vi "mop&inc.vi"() -> ()   [LabVIEW 2017]
panel:
  in  "子面板传来-开始测试":bool
  out "设备编号 2":string
  out "测试方式 2":enum32{"手动测试", "自动测试"}(ring)
  out "连接ID":refnum<k5>
  out "网络连接指示":bool
  in  "每次数据量":i32
  out "当前时间":string
  out "用户":string
  out "设备编号":dbl
  out "测试编号":dbl
  out "测试类型":dbl
  out "测试批次":dbl
  # "测试信息"
  # "根据测试类型\n和手/自动；决定\n子面板显示manual\n和auto页。manual分\nmop-manual和\ninc-manual，各功能\n按钮就是各子模块。\nauto有\n测试项（子模块）\n配置选项页。"
  # "登录信息显示"
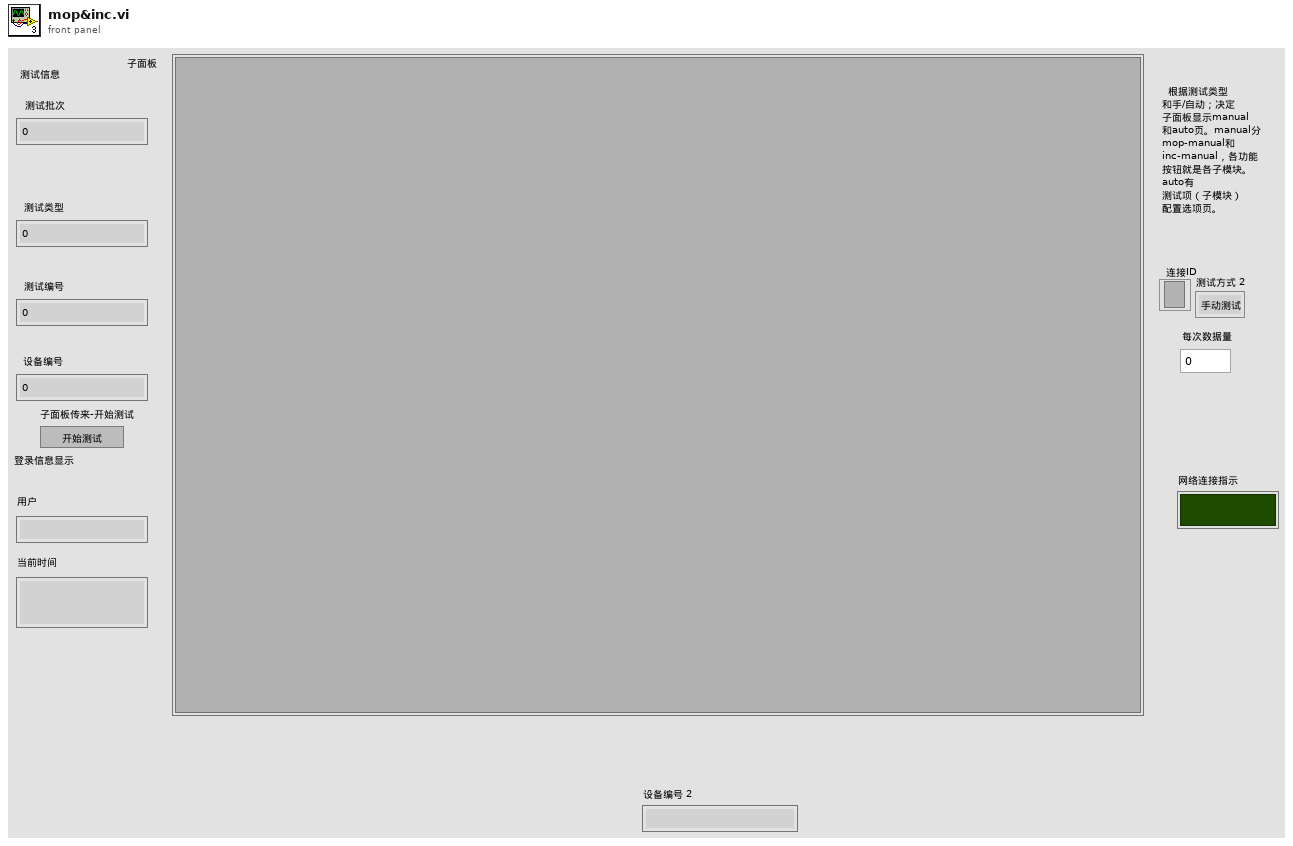
[diagram p1: front panel]
types:
  T1 = typedef "自定义枚举指令器.ctl" = enum16{"初始化", "等待用户事件", "新建测试", "用户管理"}
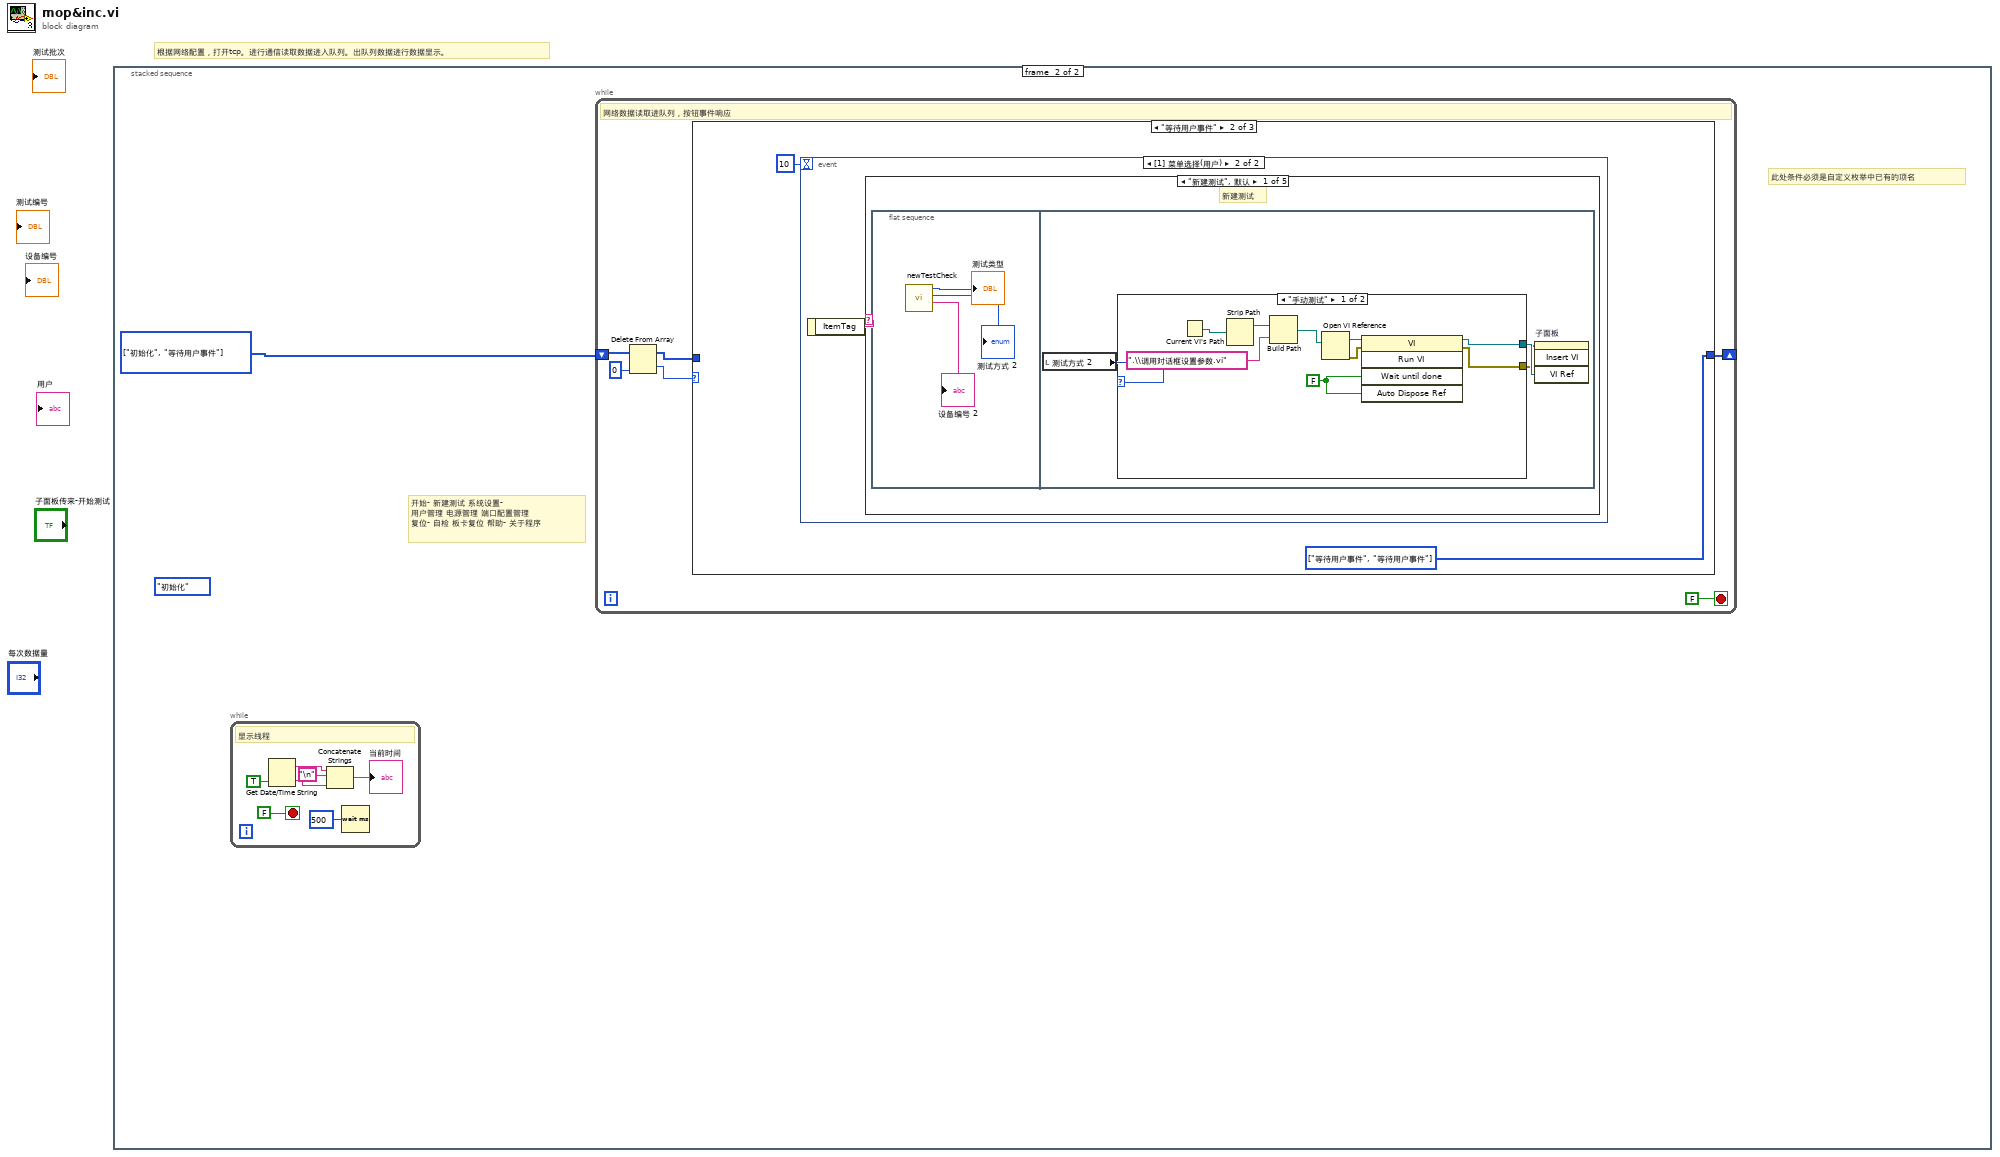
[diagram p0: block diagram]
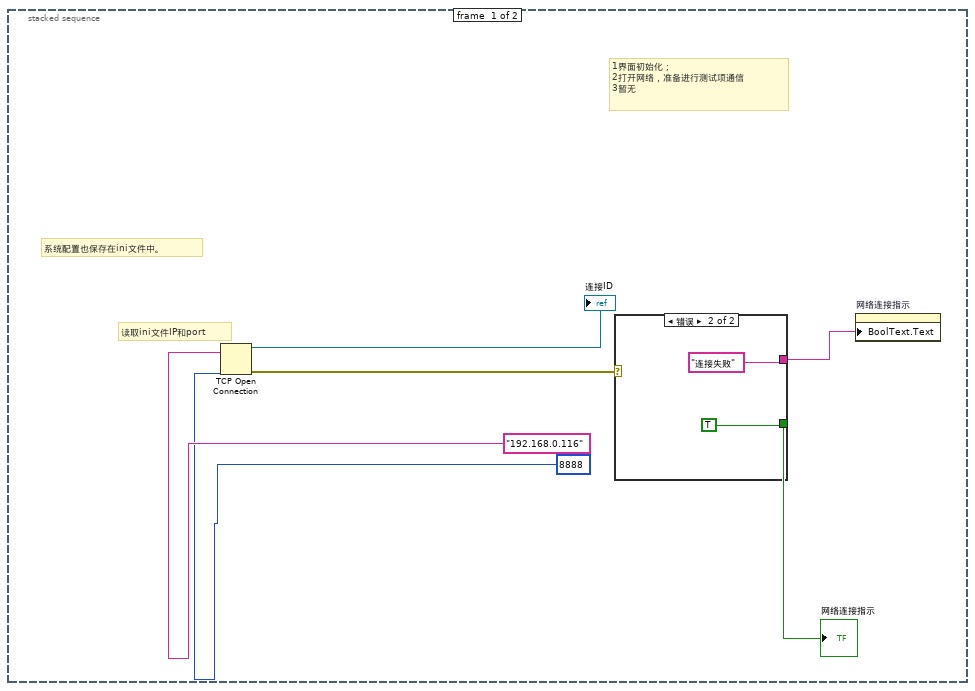
[diagram p2: hidden frame]
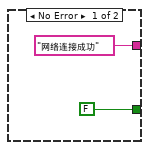
[diagram p3: hidden frame]
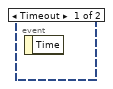
[diagram p5: hidden frame]
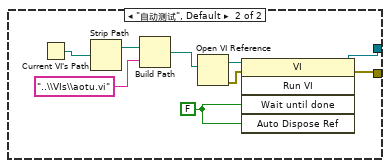
[diagram p6: hidden frame]
diagram:
  # "根据网络配置，打开tcp。进行通信读取数据进入队列。出队列数据进行数据显示。"
  n1 = stacked-sequence {
    frame #0 {
      # "读取ini文件IP和port"
      # "系统配置也保存在ini文件中。"
      # "1界面初始化；\n2打开网络，准备进行测试项通信\n3暂无"
      n2 = TCP Open Connection(address="192.168.0.116" ("地址"), remote port or service name=u16 8888 ("远程端口或服务名称")) -> (connection ID=→"连接ID":refnum<k5>, error out=w6:errorcluster)  [unwired: 3 in]
      n3 = case shown="错误" w6 {
        tunnel: [FALSE TRUE] -> w5
        tunnel: ["网络连接成功" "连接失败"] -> w4
        frame No Error {
        }
        frame Error {
        }
      }
      "网络连接指示" <- w5
      n4 = property on="网络连接指示" class="Bool (严格)"("BoolText.Text"=w4) -> ()  [unwired: 2 in, 2 out]
    }
    frame #1 {
      (unwired) 自定义枚举指令器."初始化"
      w11 = T1[] [enum."初始化", enum."等待用户事件"] items=["初始化", "等待用户事件", "新建测试", "用户管理"]
      # "开始- 新建测试 系统设置- \n用户管理 电源管理 端口配置管理 \n复位- 自检 板卡复位 帮助- 关于程序"
      # "此处条件必须是自定义枚举中已有的项名"
      n5 = while {
        stop <- FALSE stop-if-true
        # "显示线程"
        n6 = Get Date/Time String(want seconds? (F)=TRUE ("需要秒？(F)")) -> (date string=w50:string, time string=w49:string)  [unwired: 2 in]
        n7 = Concatenate Strings(w50, "\n", w49) -> (→"当前时间":string)
        n8 = Wait (ms)(milliseconds to wait=u32 500 ("等待时间（毫秒）")) -> ()  [unwired: 1 out]
      }
      n9 = while {
        shift-right: [w13] -> _
        shift-left: w11 -> [w17]
        stop <- FALSE stop-if-true
        # "网络数据读取进队列，按钮事件响应"
        n10 = Delete From Array(array=w17, index=0 ("索引")) -> (deleted portion=w15:T1, array with subset deleted=w14:T1[])  [unwired: 1 in]
        n11 = case shown="\"等待用户事件\"" w15 {
          tunnel: w14 -> [w18 _ w46]
          tunnel: [w18 w20 w46] -> w13
          frame "初始化", Default {
            # "初始化LV2数据"
          }
          frame "等待用户事件" {
            w20 = T1[] [enum."等待用户事件", enum."等待用户事件"] items=["初始化", "等待用户事件", "新建测试", "用户管理"]
            n12 = event shown="[1] 菜单选择(用户)" {
              selector: _ -> [_ _]
              dyn-events: _ -> [_ _]
              timeout: 10 -> [_ _]
              event Timeout {
                n13 = event-data() -> ()  [unwired: 1 in, 1 out]
              }
              event Menu Selection (User) {
                n14 = event-data() -> ("ItemTag"=w21:string)  [unwired: 1 in]
                n15 = case shown="\"新建测试\", 默认" w21 {
                  frame "新建测试", Default {
                    # "新建测试"
                    n16 = flat-sequence {
                      frame #0 {
                        n17 = call "newTestCheck.vi"() -> ("设备编号 2"=→"设备编号 2":string, "测试方式 2"=→"测试方式 2":enum32{"手动测试", "自动测试"}, "测试类型 2"=→"测试类型":enum32{"INC", "MOP"})  [unwired: 9 in]
                      }
                      frame #1 {
                        n18 = local read "测试方式 2"() -> (w27:enum32{"手动测试", "自动测试"})
                        n19 = case shown="\"手动测试\"" w27 {
                          tunnel: [w28 w38] -> w25
                          tunnel: [w29 w37] -> w26
                          frame "手动测试" {
                            w30 = FALSE
                            n20 = Current VI's Path() -> (path=w36:path)
                            n21 = Strip Path(path=w36) -> (stripped path=w35:path)  [unwired: 1 out]
                            n22 = Build Path(base path=w35, name or relative path=".\\调用对话框设置参数.vi" ("名称或相对路径")) -> (appended path=w33:path)
                            n23 = Open VI Reference(vi path=w33) -> (vi reference=w32:refnum<vi>, error out=w31:errorcluster)  [unwired: 5 in]
                            n24 = invoke class="VI" method="Run VI"(reference=w32, error in=w31, "Wait until done"=w30, "Auto Dispose Ref"=w30) -> (reference out=w29:refnum<vi>, error out=w28:errorcluster)  [unwired: 1 in, 3 out]
                          }
                          frame "自动测试", Default {
                            w39 = FALSE
                            n25 = Current VI's Path() -> (path=w45:path)
                            n26 = Strip Path(path=w45) -> (stripped path=w44:path)  [unwired: 1 out]
                            n27 = Build Path(base path=w44, name or relative path="..\\VIs\\aotu.vi" ("名称或相对路径")) -> (appended path=w42:path)
                            n28 = Open VI Reference(vi path=w42) -> (vi reference=w41:refnum<vi>, error out=w40:errorcluster)  [unwired: 5 in]
                            n29 = invoke class="VI" method="Run VI"(reference=w41, error in=w40, "Wait until done"=w39, "Auto Dispose Ref"=w39) -> (reference out=w37:refnum<vi>, error out=w38:errorcluster)  [unwired: 1 in, 3 out]
                          }
                        }
                        n30 = invoke on="子面板" class="SubPnl" method="Insert VI"(error in=w25, "VI Ref"=w26) -> ()  [unwired: 2 in, 4 out]
                      }
                    }
                  }
                  frame "用户管理" {
                  }
                  frame "电源管理" {
                  }
                  frame "端口配置管理" {
                  }
                  frame "自检" {
                  }
                }
              }
            }
          }
          frame "新建测试" {
            # "此处条件必须是自定义枚举中已有的项名，事件1--是暂时测试使用"
          }
        }
      }
    }
  }
